vi "Main.vi"() -> ()   [LabVIEW 2026]
doc: "VI TIMESTAMP — DOCUMENTATION\n============================\nInstitut Fresnel | USB-6353 | CTR3 | PFI7 | 100 MHz | LabVIEW 2025\n\n\nOBJECTIF\n--------\nEnregistrer le timestamp absolu de chaque trigger caméra avec une\nprécision hardware de 10 ns. Résultat écrit dans un fichier CSV,\nécrasé à chaque nouvelle acquisition.\n\n\nPRINCIPE\n--------\nCTR3 compte les ticks de l'horloge interne 100 MHz. Le signal trigger\n(P0.4, rebouclé sur PFI7) est l'horloge d'échantillonnage : à chaque\nflanc montant, CTR3 capture la valeur courante du compteur.\n\n T_absolu = T0 + (ticks + offset_rollover) / 100 000 000\n\nT0 = heure système au démarrage (Get Date/Time In Seconds).\noffset_rollover = compensation du débordement 32 bits (rollover ~42.9 s).\n\n\nMACHINE À ÉTATS\n---------------\nIDLE ? INIT ? START ? RUNNING ? WRITE ? STOP ? IDLE\n\n IDLE : attente bouton Start, lecture N (nb frames)\n INIT : création tâche CTR3, config timing PFI7, ouverture CSV, T0\n START : DAQmx Start Task — doit précéder les tâches DO/AO du VI principal\n RUNNING : DAQmx Read non-bloquant (timeout 0.01 s) — boucle sur lui-même\n WRITE : calcul timestamp, gestion rollover, écriture ligne CSV\n STOP : Stop Task, Clear Task, Close File, reset SR\n\n\nGESTION ROLLOVER (dans WRITE)\n------------------------------\n Si ticks < ticks_prev ? offset += 4 294 967 296\n ticks_prev ? ticks (valeur brute, sans offset)\n\n\nSHIFT REGISTERS\n---------------\n état Enum État courant\n task ref DAQmx Task Référence CTR3\n file ref File Refnum Fichier CSV ouvert\n T0 Timestamp Heure au Start\n ticks DBL Valeur DAQmx Read\n ticks_prev DBL (init 0) Ticks de la frame précédente\n offset DBL (init 0) Cumul rollovers × 2^32\n frame_i I32 (init 0) Index frame courante\n\n\nFORMAT CSV\n----------\n frame_index I32 Index frame (0-indexé)\n timestamp_iso String Ex : 2026-03-09T11:13:54.223 (ISO 8601)\n timestamp_unix DBL Ex : 3855896034.224 (secondes depuis 01/01/1904)\n\nConversion Python :\n df['datetime'] = pd.to_datetime(df['timestamp_unix'] - 2082844800, unit='s')\n\n\nVALIDATION\n----------\n 20.9 Hz jitter 358 µs (vient du générateur NI-MAX, pas du VI) ?\n 0.1 Hz 2 rollovers détectés et compensés, monotonie OK ?"
uses:
  controls/State.ctl
  controls/TypeDef_FGV.ctl
  <vilib>/DAQmx/read.llb/DAQmx Read (Counter DBL 1Chan 1Samp).vi
  <vilib>/DAQmx/create/channels.llb/DAQmx Create Channel (CI-Count Edges).vi
  <vilib>/DAQmx/configure/timing.llb/DAQmx Timing (Sample Clock).vi
  <vilib>/DAQmx/miscellaneous.llb/DAQmx Fill In Error Info.vi
  <vilib>/Utility/file.llb/Write Delimited Spreadsheet (DBL).vi
  <resource>/objmgr/daqmx.rc
  <userlib>/_OpenG.lib/error/error.llb/openg_error.lvlib
panel:
  in  "file path (dialog if empty)":path
  out "output array":dbl[](array[numeric])
  out "x >= y?":bool
  out "frame_i":i32
  in  "file path":path=path "C:/Users/spinning polar/Desktop/TRASH/Timestamp.csv"
  in  "samples per channel":i32=10 caption="échantillons par voie"
  in  "Stop":bool
  in  "Start":bool
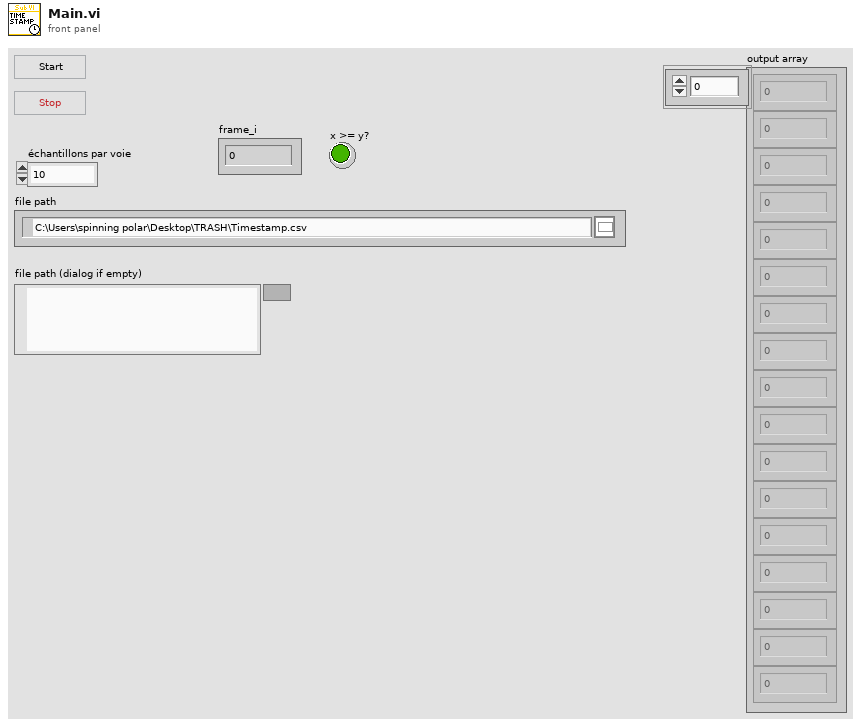
[diagram p1: front panel]
types:
  T1 = typedef "State.ctl" = enum16{"IDLE", "INIT", "START", "RUNNING", "WRITE", "STOP"}
  T2 = typedef "TypeDef_FGV.ctl" = enum16{"Initialize", "Add", "Read"}
  T3 = enum16{"open", "replace", "create", "open or create", "replace or create", "replace or create with confirmation"}
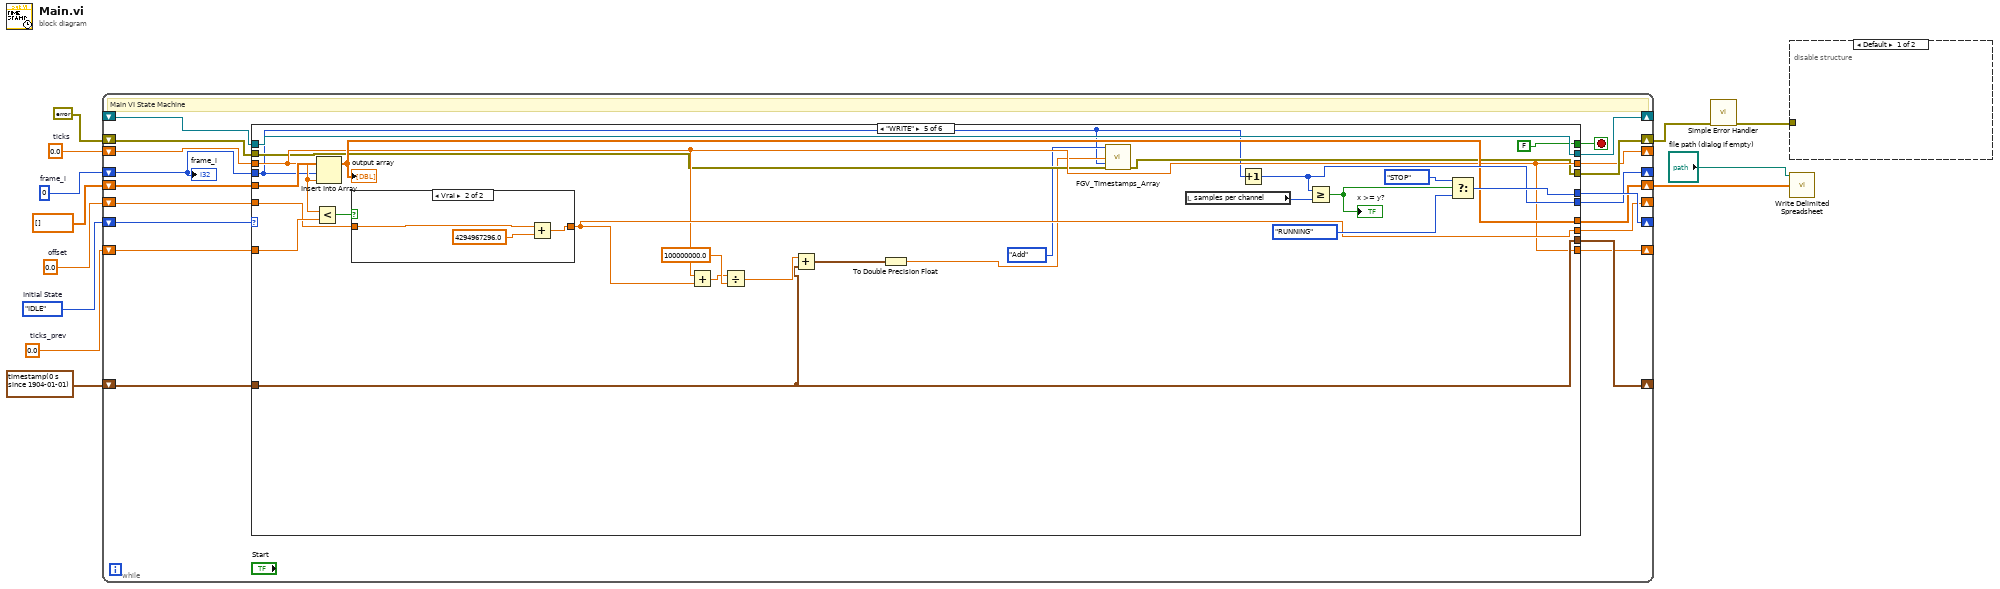
[diagram p0: block diagram]
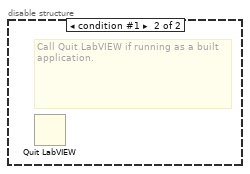
[diagram p2: hidden frame]
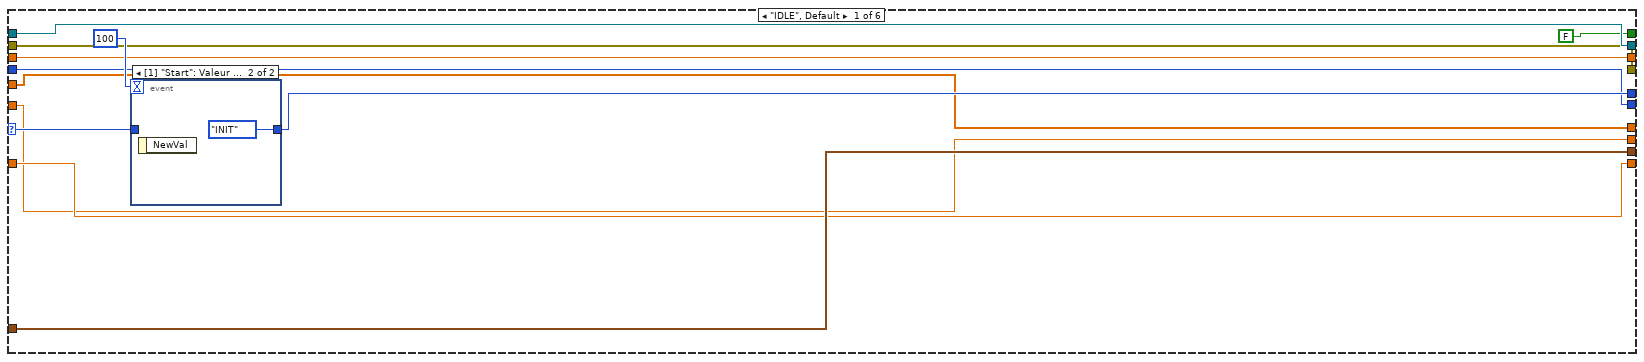
[diagram p3: hidden frame]
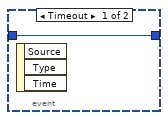
[diagram p4: hidden frame]
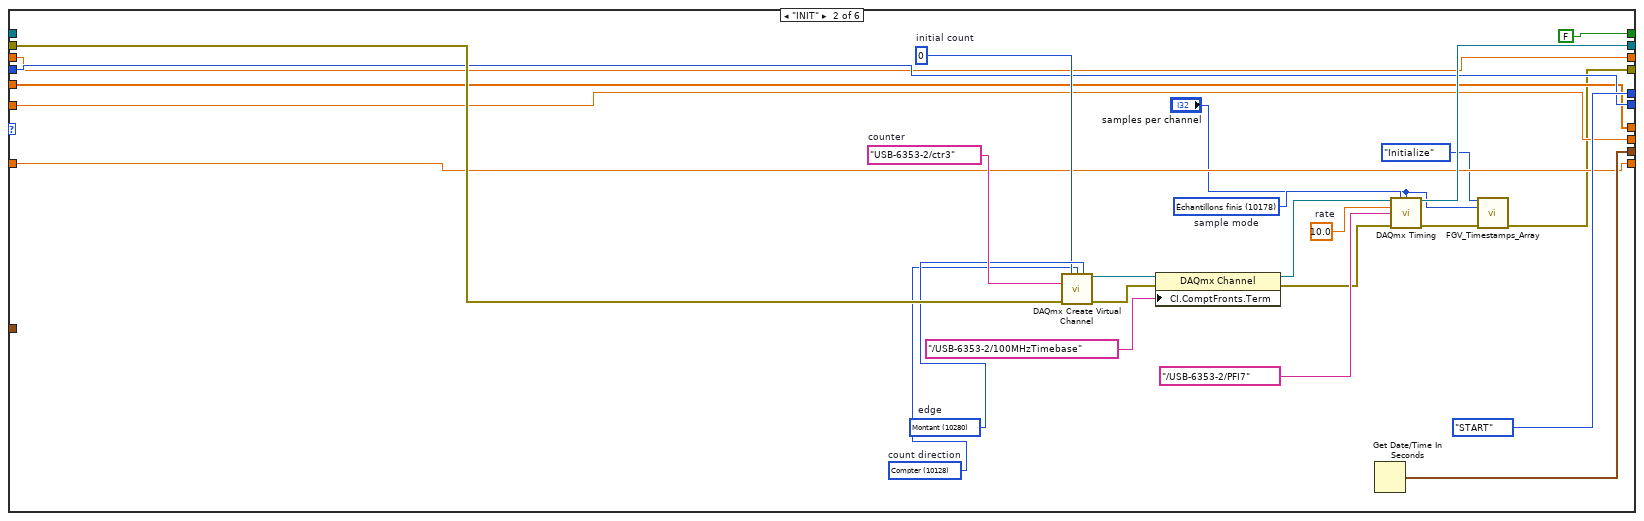
[diagram p5: hidden frame]
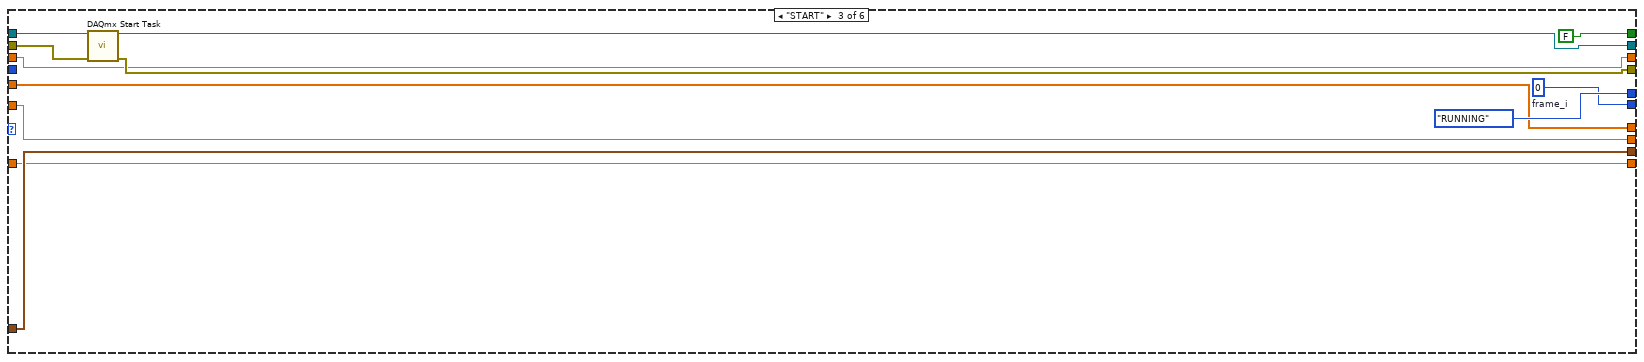
[diagram p6: hidden frame]
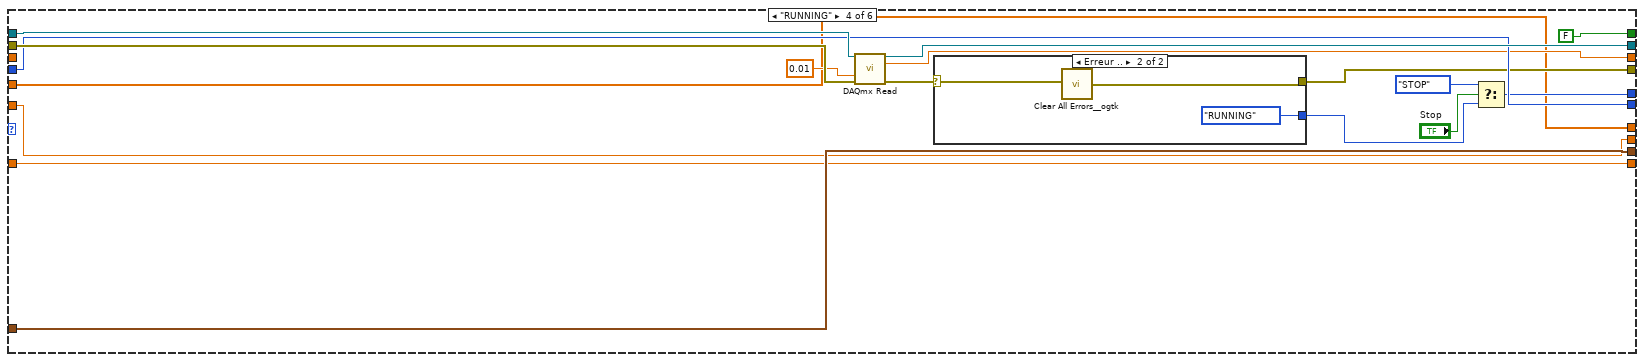
[diagram p7: hidden frame]
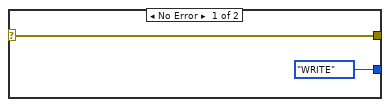
[diagram p8: hidden frame]
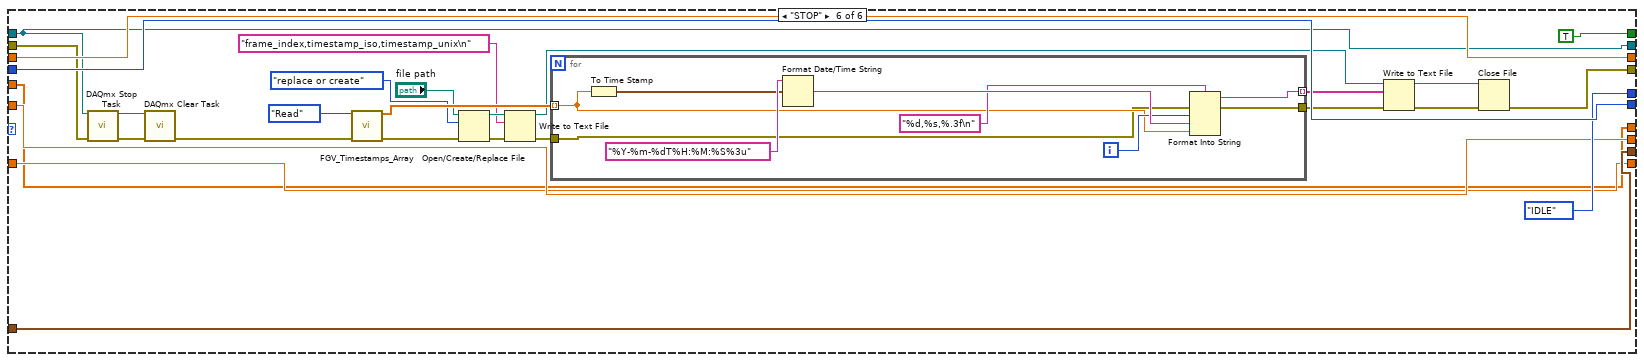
[diagram p10: hidden frame]
diagram:
  w5 = 0.0  # offset
  w4 = 0.0  # ticks_prev
  w7 = 0.0  # ticks
  w8 = 0  # frame_i
  w12 = State."IDLE"  # Initial State
  n1 = while {
    shift-right: [w30] -> _
    shift-left: w12 -> [w31]
    shift-right: [w28] -> w10
    shift-left: errorcluster {"status"=FALSE, "code"=0, "source"=""} ("error constant") -> [w29]
    shift-right: [w27] -> _
    shift-left: _ -> [w26]
    shift-right: [w25] -> _
    shift-left: timestamp(0 s since 1904-01-01) ("seconds since 1Jan1904") -> [w24]
    shift-right: [w23] -> _
    shift-left: w8 -> [w22]
    shift-right: [w20] -> _
    shift-left: w7 -> [w19]
    shift-right: [w16] -> _
    shift-left: w5 -> [w15]
    shift-right: [w18] -> _
    shift-left: w4 -> [w17]
    shift-right: [w14] -> w2
    shift-left: dbl[] [] -> [w13]
    stop <- w21 stop-if-true
    # "Main VI State Machine"
    n2 = case shown="\"WRITE\"" w31 {
      selector: w31 -> [w41 _ _ _ _ _]
      tunnel: [w42 State."START" ("Initial State") State."RUNNING" ("Initial State") w88 w122 State."IDLE" ("Initial State")] -> w30
      tunnel: w29 -> [w39 w71 w80 w99 w110 w154]
      tunnel: [w39 w48 w77 w92 w109 w153] -> w28
      tunnel: [w40 w65 w78 w98 w130 w156] -> w27
      tunnel: w26 -> [w40 _ w81 w100 w130 w156]
      tunnel: [w38 w63 w83 w96 w127 w160] -> w25
      tunnel: w24 -> [w38 _ w83 w96 w127 w160]
      tunnel: [w37 w55 w79 w97 w116 w161] -> w23
      tunnel: w22 -> [w37 w55 _ w97 w106 w161]
      tunnel: [FALSE ("Stop") FALSE ("Stop") FALSE ("Stop") FALSE ("Stop") FALSE ("Stop") TRUE ("Stop")] -> w21
      tunnel: [w35 w53 w75 w94 w111 w158] -> w20
      tunnel: w19 -> [w35 w53 w75 _ w111 w158]
      tunnel: [w34 w52 w74 w85 w111 w151] -> w18
      tunnel: w17 -> [w34 w52 w74 w85 w119 w151]
      tunnel: [w33 w51 w73 w86 w112 w152] -> w16
      tunnel: w15 -> [w33 w51 w73 w86 w117 w152]
      tunnel: [w32 w50 w72 w84 w115 w150] -> w14
      tunnel: w13 -> [w32 w50 w72 w84 w114 w150]
      frame "IDLE", Default {
        n3 = event shown="[1] \"Start\": Valeur changée" {
          selector: _ -> [_ _]
          dyn-events: _ -> [_ _]
          timeout: 100 -> [_ _]
          tunnel: [w44 State."INIT" ("Initial State")] -> w42
          tunnel: w41 -> [w44 _]
          event Timeout {
            n4 = event-data() -> ()  [unwired: 1 in, 3 out]
          }
          event "Start": Value Change {
            n5 = event-data() -> ()  [unwired: 1 in, 1 out]
          }
        }
      }
      frame "INIT" {
        w61 = 10.0  # rate
        w64 = 10178 items=["Échantillons finis"=10178, "Échantillons continus"=10123, "Point par point avec cadencement matériel"=12522]  # sample mode
        w66 = 10128 items=["Compter"=10128, "Compter à rebours"=10124, "Contrôlé de manière externe"=10326]  # count direction
        w67 = u32 0  # initial count
        w68 = 10280 items=["Montant"=10280, "Descendant"=10171]  # edge
        w69 = tag "USB-6353-2/ctr3"  # counter
        n6 = call-poly <vilib>:"DAQmx Create Virtual Channel.vi"("initial count"=w67, "count direction"=w66, "edge"=w68, "counter"=w69, "error in"=w71) -> ("task out"=w59:refnum<k21>, "error out"=w60:errorcluster)  [unwired: 9 in]
        n7 = property class="DAQmx Channel"(reference=w59, error in=w60, "CI.ComptFronts.Term"=tag "/USB-6353-2/100MHzTimebase") -> (reference out=w58:refnum<k21>, error out=w57:errorcluster)
        n8 = Get Date/Time In Seconds() -> (seconds since 1Jan1904=w63:timestamp)
        n9 = call-poly <vilib>:"DAQmx Timing.vi"("task/channels in"=w58, "sample mode"=w64, "samples per channel"="samples per channel", "rate"=w61, "source"=tag "/USB-6353-2/PFI7", "error in"=w57) -> ("task out"=w65:refnum<k21>, "error out"=w49:errorcluster)  [unwired: 8 in]
        n10 = call "FGV_Timestamps_Array.vi"("Action"=TypeDef_FGV."Initialize", "Size"="samples per channel", "error in"=w49) -> ("error out"=w48:errorcluster)  [unwired: 11 in, 1 out]
      }
      frame "START" {
        w79 = 0  # frame_i
        n11 = call <vilib>:"DAQmx Start Task.vi"("task/channels in"=w81, "error in"=w80) -> ("task out"=w78:refnum<k21>, "error out"=w77:errorcluster)  [unwired: 12 in]
      }
      frame "RUNNING" {
        n12 = call-poly <vilib>:"DAQmx Read.vi"("task/channels in"=w100, "timeout"=0.01, "error in"=w99) -> ("task out"=w98:refnum<k21>, "data"=w94:dbl, "error out"=w93:errorcluster)  [unwired: 10 in]
        n13 = case shown="Erreur .." w93 {
          selector: w93 -> [w101 w104]
          tunnel: [State."WRITE" ("Initial State") State."RUNNING" ("Initial State")] -> w90
          tunnel: [w101 w103] -> w92
          frame No Error {
          }
          frame Error {
            n14 = call <userlib>:"Clear All Errors__ogtk.vi"("Error In"=w104) -> ("Error Out"=w103:errorcluster)  [unwired: 3 in]
          }
        }
        n15 = Select(t=State."STOP" ("Initial State"), s="Stop", f=w90) -> (s? t:f=w88:T1)
      }
      frame "WRITE" {
        n16 = Less?(x=w111, y=w119) -> (x < y?=w118:bool)
        n17 = Insert Into Array(array=w114, index=w106, new element=w111) -> (w115:dbl[])
        "output array" <- w115
        n18 = case shown="Vrai" w118 {
          tunnel: w117 -> [w131 w133]
          tunnel: [w131 w132] -> w112
          frame False {
          }
          frame True {
            n19 = Add(x=w133, y=4294967296.0) -> (x+y=w132:dbl)
          }
        }
        n20 = Add(x=w111, y=w112) -> (x+y=w113:dbl)
        n21 = Divide(x=w113, y=100000000.0) -> (x/y=w128:dbl)
        n22 = Add(x=w128, y=w127) -> (x+y=w126:timestamp)
        n23 = To Double Precision Float(number=w126) -> (double precision float=w107:dbl)
        n24 = call "FGV_Timestamps_Array.vi"("Action"=TypeDef_FGV."Add", "Value to add"=w107, "Index"=w106, "error in"=w110) -> ("error out"=w109:errorcluster)  [unwired: 10 in, 1 out]
        n25 = local read "samples per channel"() -> (w125:i32)
        n26 = Increment(x=w106) -> (x+1=w116:i32)
        n27 = Greater Or Equal?(x=w116, y=w125) -> (x >= y?=w121:bool)
        "x >= y?" <- w121
        n28 = Select(t=State."STOP" ("Initial State"), s=w121, f=State."RUNNING" ("Initial State")) -> (s? t:f=w122:T1)
      }
      frame "STOP" {
        n29 = call <vilib>:"DAQmx Stop Task.vi"("task/channels in"=w156, "error in"=w154) -> ("task out"=w157:refnum<k21>, "error out"=w155:errorcluster)  [unwired: 12 in]
        n30 = call <vilib>:"DAQmx Clear Task.vi"("task in"=w157, "error in"=w155) -> ("error out"=w149:errorcluster)  [unwired: 13 in]
        n31 = call "FGV_Timestamps_Array.vi"("Action"=TypeDef_FGV."Read", "error in"=w149) -> ("Timestamps_Array OUT"=w147:dbl[], "error out"=w139:errorcluster)  [unwired: 12 in]
        n32 = Open/Create/Replace File(file path (use dialog)="file path", error in=w139, operation (0:open)=T3."replace or create") -> (refnum out=w142:refnum<file>, error out=w143:errorcluster)  [unwired: 3 in, 1 out]
        n33 = Write to Text File(file (use dialog)=w142, text="frame_index,timestamp_iso,timestamp_unix\n", error in=w143) -> (refnum out=w135:refnum<file>, error out=w138:errorcluster)  [unwired: 1 in, 1 out]
        n34 = for {
          tunnel: w147 -> [w166] mode=indexing
          tunnel: w138 -> [w165]
          tunnel: [w164] -> w146
          tunnel: [w163] -> w145 mode=indexing
          i -> [w167]
          n35 = To Time Stamp(1:w166) -> (0:w168:timestamp)
          n36 = Format Date/Time String(time format string (%c)="%Y-%m-%dT%H:%M:%S%3u", seconds (now)=w168) -> (date/time string=w171:string)  [unwired: 1 in]
          n37 = Format Into String(format string="%d,%s,%.3f\n", error in=w165, w167, w171, w166) -> (resulting string=w163:string, error out=w164:errorcluster)  [unwired: 1 in]
        }
        n38 = Write to Text File(file (use dialog)=w135, text=w145, error in=w146) -> (refnum out=w136:refnum<file>, error out=w137:errorcluster)  [unwired: 1 in, 1 out]
        n39 = Close File(refnum=w136, error in=w137) -> (error out=w153:errorcluster)  [unwired: 1 out]
      }
    }
    "frame_i" <- w22
  }
  n40 = call <vilib>:"Simple Error Handler.vi"("error in (no error)"=w10) -> ("error out"=w9:errorcluster)  [unwired: 4 in, 4 out]
  n41 = disable-structure shown="Default" {
    disable-tunnel: w9 -> [_ _]
    frame condition #0 (active) {
    }
    frame condition #1 {
      # "Call Quit LabVIEW if running as a built application."
      n42 = Quit LabVIEW() -> ()  [unwired: 1 in]
    }
  }
  n43 = call-poly <vilib>:"Write Delimited Spreadsheet.vi"("file path (dialog if empty)"="file path (dialog if empty)", "1D data"=w2) -> ()  [unwired: 12 in, 2 out]
